vi "main.vi"() -> (5 "control":i32)   [LabVIEW 2014]
uses:
  <vilib>/Utility/miscctls.llb/LVPositionTypeDef.ctl
  Control 1.ctl
panel:
  out "Player2 energy":dbl
  out "Player1 skill":u8(slide) scale=0.0..100.0
  out "stop":bool
  out "Time(s)":dbl
  out "deliver2":T1
  out "deliver":T1
  out "player2":bool
  out "Position 2":T2
  out "control 2":i32
  out "test 2":i16
  out "player1":bool
  out "Position":T2
  out "test":i16
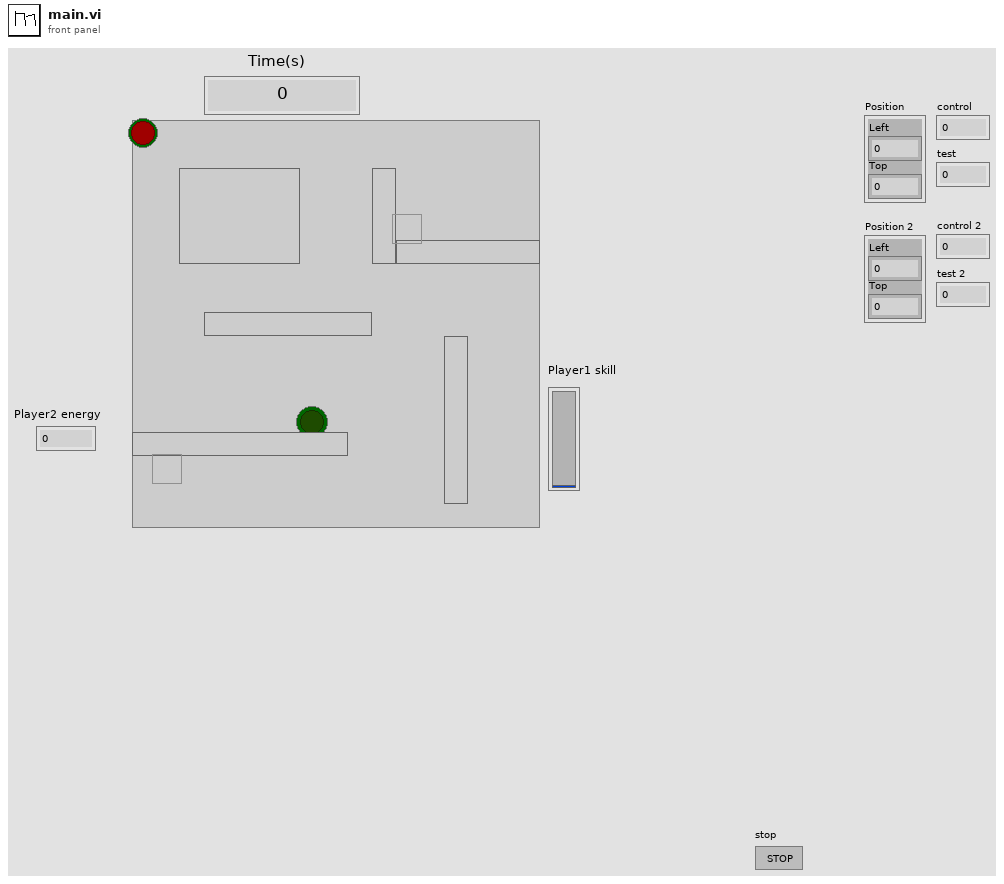
[diagram p1: front panel]
types:
  T1 = typedef "Control 1.ctl" = bool
  T2 = typedef "LVPositionTypeDef.ctl" = cluster{"Left":i32, "Top":i32}
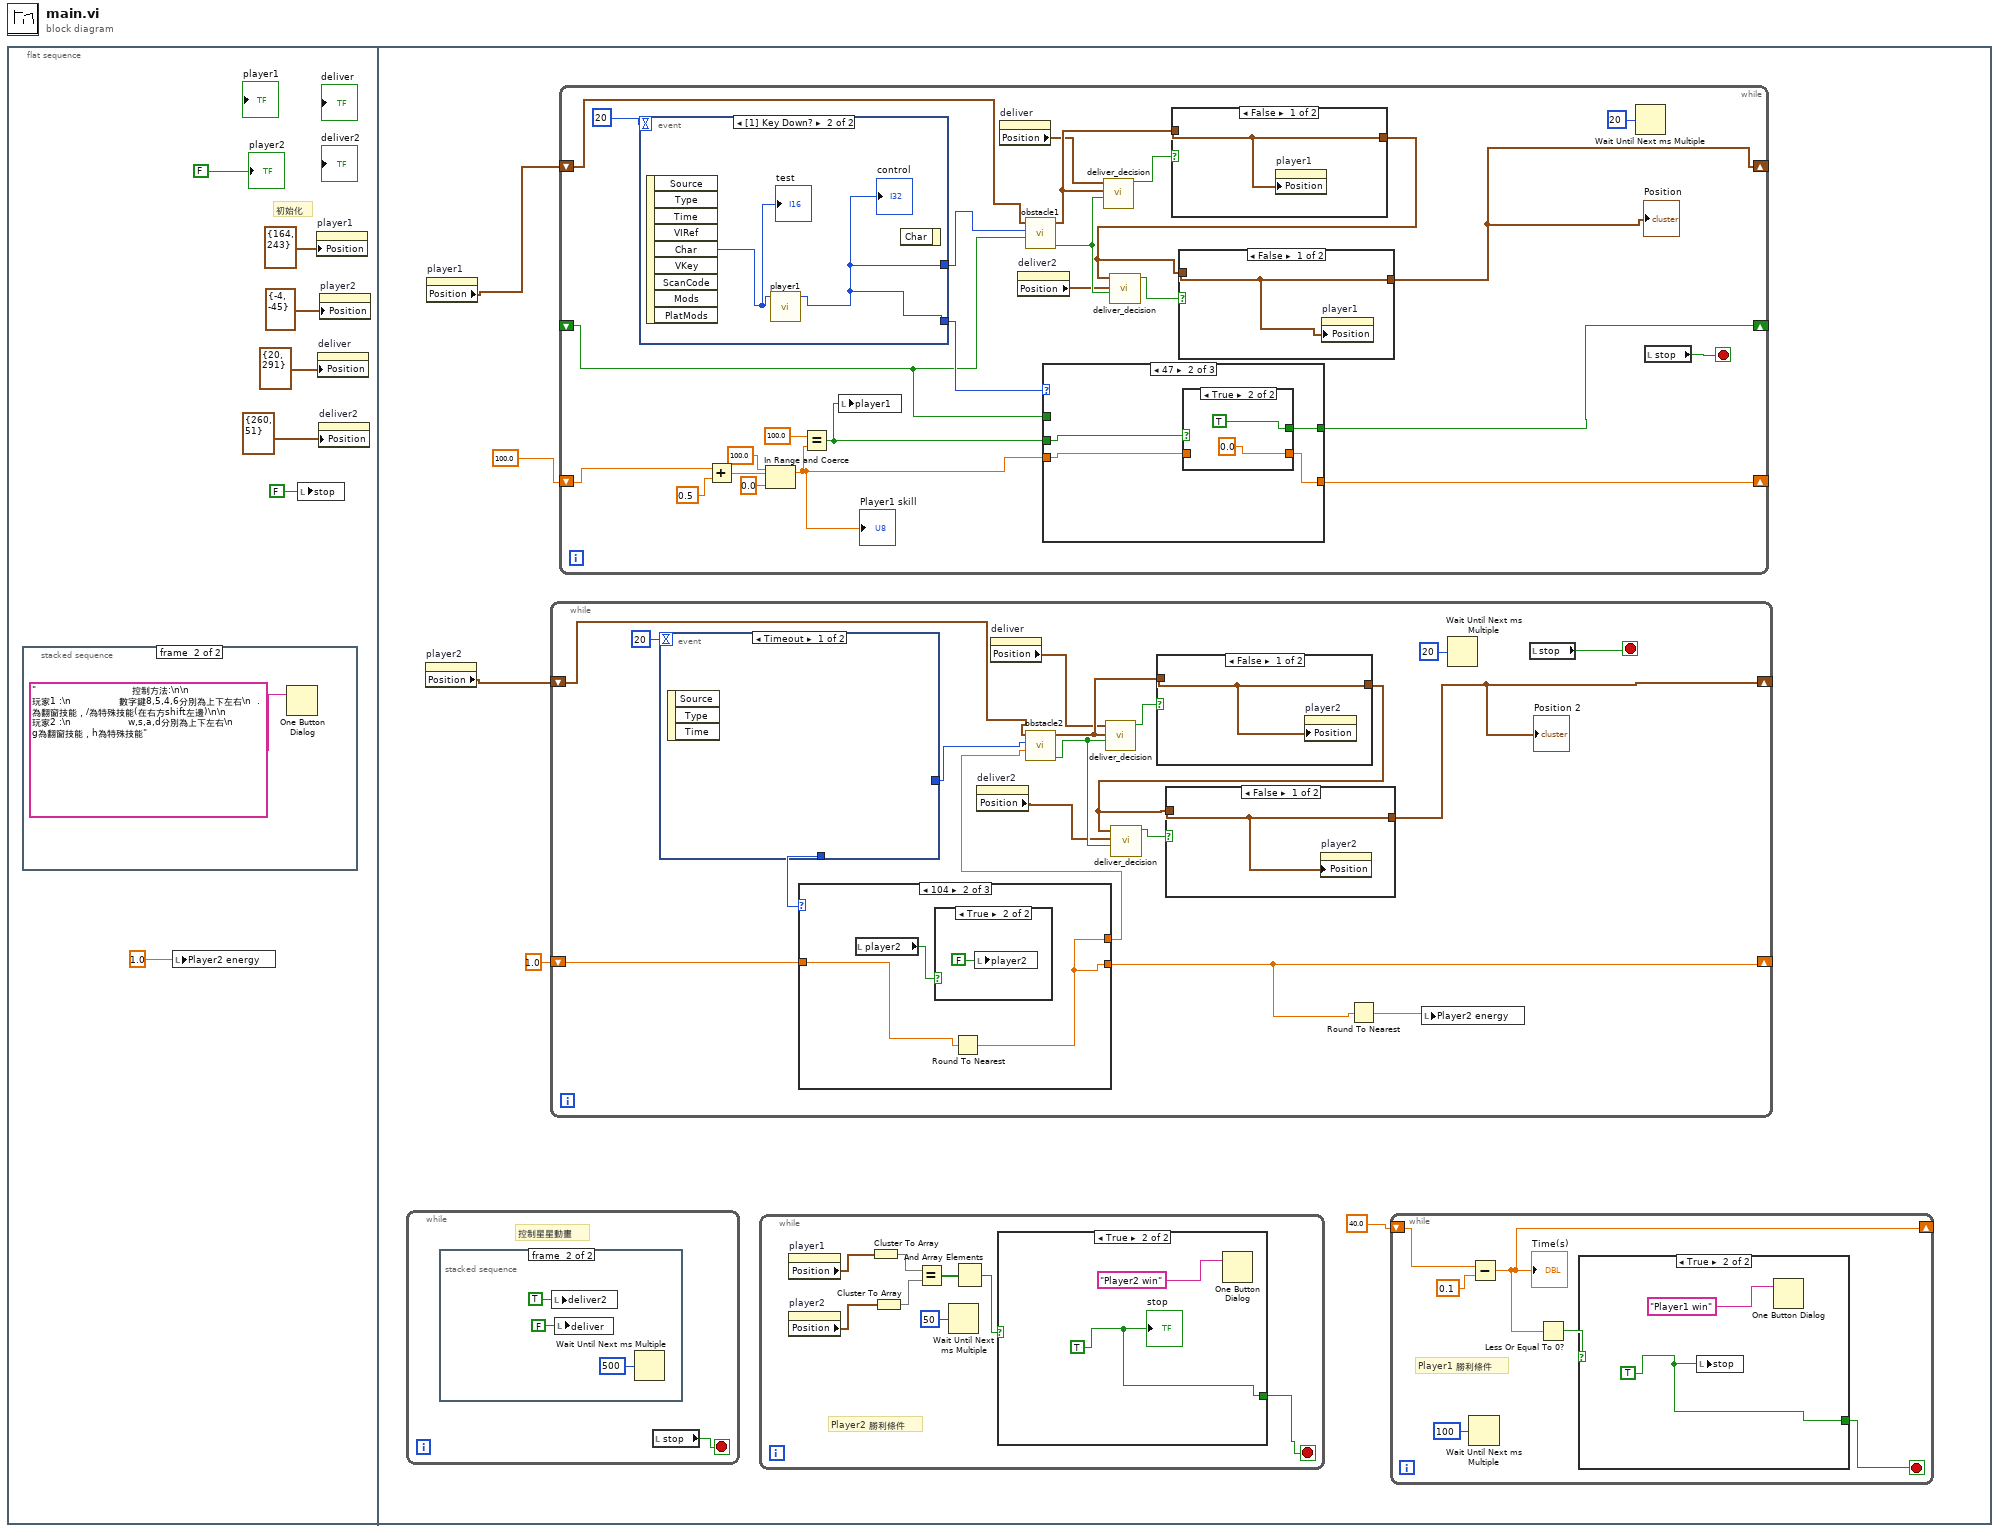
[diagram p0: block diagram]
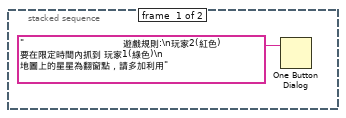
[diagram p2: hidden frame]
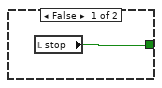
[diagram p3: hidden frame]
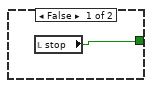
[diagram p4: hidden frame]
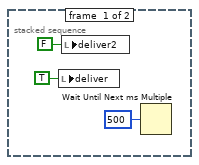
[diagram p5: hidden frame]
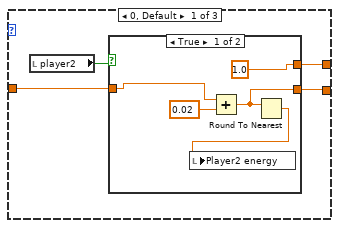
[diagram p6: hidden frame]
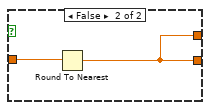
[diagram p7: hidden frame]
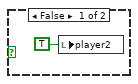
[diagram p8: hidden frame]
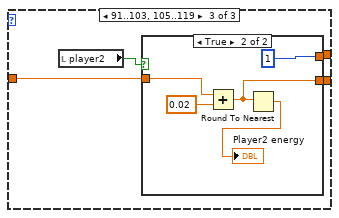
[diagram p9: hidden frame]
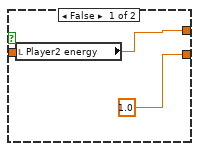
[diagram p10: hidden frame]
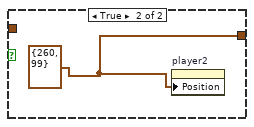
[diagram p11: hidden frame]
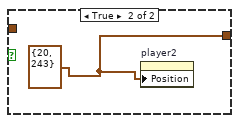
[diagram p12: hidden frame]
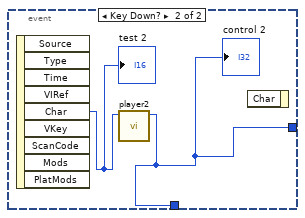
[diagram p13: hidden frame]
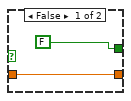
[diagram p15: hidden frame]
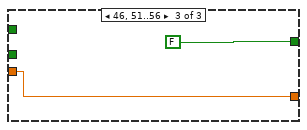
[diagram p16: hidden frame]
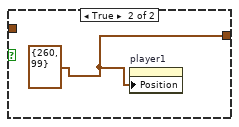
[diagram p17: hidden frame]
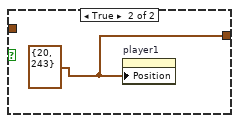
[diagram p18: hidden frame]
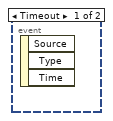
[diagram p19: hidden frame]
diagram:
  n1 = flat-sequence {
    frame #0 {
      # "初始化"
      n2 = stacked-sequence {
        frame #0 {
          n3 = One Button Dialog(message="                                 遊戲規則:\n玩家2(紅色) 要在限定時間內抓到 玩家1(綠色)\n       地圖上的星星為翻窗點，請多加利用") -> ()  [unwired: 1 in, 1 out]
        }
        frame #1 {
          n4 = One Button Dialog(message="                                控制方法:\n\n                                   玩家1 :\n                數字鍵8,5,4,6分別為上下左右\n  .為翻窗技能，/為特殊技能(在右方shift左邊)\n\n                                  玩家2 :\n                   w,s,a,d分別為上下左右\n               g為翻窗技能，h為特殊技能") -> ()  [unwired: 1 in, 1 out]
        }
      }
      n5 = local write "Player2 energy"(1.0 ("energy")) -> ()
      n6 = local write "stop"(FALSE ("stop 4")) -> ()
      n7 = property on="player1" class="Bool (strict)"("Position"=T2 {"Left"=164, "Top"=243}) -> ()  [unwired: 2 in, 2 out]
      n8 = property on="deliver" class="Bool (strict)"("Position"=T2 {"Left"=20, "Top"=291}) -> ()  [unwired: 2 in, 2 out]
      n9 = property on="deliver2" class="Bool (strict)"("Position"=T2 {"Left"=260, "Top"=51}) -> ()  [unwired: 2 in, 2 out]
      n10 = property on="player2" class="Bool (strict)"("Position"=T2 {"Left"=-4, "Top"=-45}) -> ()  [unwired: 2 in, 2 out]
      "player2" <- FALSE
    }
    frame #1 {
      n11 = while {
        stop <- w35 stop-if-true
        # "控制星星動畫"
        n12 = stacked-sequence {
          frame #0 {
            n13 = local write "deliver"(T1 TRUE ("deliver")) -> ()
            n14 = local write "deliver2"(T1 FALSE ("deliver2")) -> ()
            n15 = Wait Until Next ms Multiple(millisecond multiple=u32 500) -> ()  [unwired: 1 out]
          }
          frame #1 {
            n16 = local write "deliver2"(T1 TRUE ("deliver2")) -> ()
            n17 = local write "deliver"(T1 FALSE ("deliver")) -> ()
            n18 = Wait Until Next ms Multiple(millisecond multiple=u32 500) -> ()  [unwired: 1 out]
          }
        }
        n19 = local read "stop"() -> (w35:bool)
      }
      n20 = property on="player2" class="Bool (strict)"() -> ("Position"=w13:T2)  [unwired: 2 in, 2 out]
      n21 = property on="player1" class="Bool (strict)"() -> ("Position"=w14:T2)  [unwired: 2 in, 2 out]
      n22 = while {
        shift-right: [w51] -> _
        shift-left: w13 -> [w57]
        shift-right: [w43] -> _
        shift-left: 1.0 -> [w44]
        stop <- w48 stop-if-true
        n23 = event shown="[0] Timeout" {
          selector: _ -> [_ _]
          dyn-events: _ -> [_ _]
          timeout: 20 -> [_ _]
          tunnel: [_ w91] -> w58
          tunnel: [_ w91] -> w46
          event Timeout {
            n24 = event-data() -> ()  [unwired: 1 in, 3 out]
          }
          event Key Down? {
            n25 = event-data() -> ("Char"=w92:i16)  [unwired: 1 in, 8 out]
            "test 2" <- w92
            n26 = call "player2.vi"("Char"=w92) -> ("f"=w91:i32)  [unwired: 10 in]
            "control 2" <- w91
            n27 = event-data() -> ()  [unwired: 2 in, 1 out]
          }
        }
        n28 = case shown="104" w46 {
          tunnel: [w60 w71 w78] -> w45
          tunnel: [w62 w71 w77] -> w43
          tunnel: w44 -> [w63 w72 w76]
          frame 0, Default {
            n29 = local read "player2"() -> (w61:bool)
            n30 = case shown="True" w61 {
              tunnel: w63 -> [w67 w70]
              tunnel: [w64 w69] -> w62
              tunnel: [1.0 w69] -> w60
              frame True {
                n31 = Add(x=w67, y=0.02) -> (x+y=w64:dbl)
                n32 = Round To Nearest(number=w64) -> (nearest integer value=w65:dbl)
                n33 = local write "Player2 energy"(w65) -> ()
              }
              frame False {
                n34 = Round To Nearest(number=w70) -> (nearest integer value=w69:dbl)
              }
            }
          }
          frame 104 {
            n35 = local read "player2"() -> (w73:bool)
            n36 = case shown="True" w73 {
              frame False {
                n37 = local write "player2"(TRUE ("player2")) -> ()
              }
              frame True {
                n38 = local write "player2"(FALSE ("player2")) -> ()
              }
            }
            n39 = Round To Nearest(number=w72) -> (nearest integer value=w71:dbl)
          }
          frame 91..103, 105..119 {
            n40 = local read "player2"() -> (w79:bool)
            n41 = case shown="True" w79 {
              tunnel: [w81 1] -> w78
              tunnel: [1.0 w83] -> w77
              tunnel: w76 -> [_ w82]
              frame False {
                n42 = local read "Player2 energy"() -> (w81:dbl)
              }
              frame True {
                n43 = Add(x=w82, y=0.02) -> (x+y=w83:dbl)
                n44 = Round To Nearest(number=w83) -> (nearest integer value=→"Player2 energy":dbl)
              }
            }
          }
        }
        n45 = property on="deliver2" class="Bool (strict)"() -> ("Position"=w49:T2)  [unwired: 2 in, 2 out]
        n46 = property on="deliver" class="Bool (strict)"() -> ("Position"=w50:T2)  [unwired: 2 in, 2 out]
        n47 = call "obstacle2.vi"("Numeric"=w45, "f"=w58, "Position in"=w57) -> ("deliver"=w54:bool, "Position out"=w55:T2)  [unwired: 7 in]
        n48 = call "deliver_decision.vi"("deliver"=w54, "Position in"=w55, "Position"=w50) -> ("Boolean"=w56:bool)  [unwired: 8 in]
        n49 = case shown="False" w56 {
          tunnel: [w89 w90] -> w52
          tunnel: w55 -> [w89 _]
          frame False {
            n50 = property on="player2" class="Bool (strict)"("Position"=w89) -> ()  [unwired: 2 in, 2 out]
          }
          frame True {
            w90 = T2 {"Left"=20, "Top"=243} ("Position")
            n51 = property on="player2" class="Bool (strict)"("Position"=w90) -> ()  [unwired: 2 in, 2 out]
          }
        }
        n52 = call "deliver_decision.vi"("deliver"=w54, "Position in"=w49, "Position"=w52) -> ("Boolean"=w53:bool)  [unwired: 8 in]
        n53 = case shown="False" w53 {
          tunnel: [w87 w88] -> w51
          tunnel: w52 -> [w87 _]
          frame False {
            n54 = property on="player2" class="Bool (strict)"("Position"=w87) -> ()  [unwired: 2 in, 2 out]
          }
          frame True {
            w88 = T2 {"Left"=260, "Top"=99} ("Position")
            n55 = property on="player2" class="Bool (strict)"("Position"=w88) -> ()  [unwired: 2 in, 2 out]
          }
        }
        "Position 2" <- w51
        n56 = Round To Nearest(number=w43) -> (nearest integer value=w42:dbl)
        n57 = local write "Player2 energy"(w42) -> ()
        n58 = Wait Until Next ms Multiple(millisecond multiple=u32 20) -> ()  [unwired: 1 out]
        n59 = local read "stop"() -> (w48:bool)
      }
      n60 = while {
        shift-right: [w109] -> _
        shift-left: w14 -> [w116]
        shift-right: [w103] -> _
        shift-left: _ -> [w102]
        shift-right: [w101] -> _
        shift-left: 100.0 -> [w94]
        stop <- w106 stop-if-true
        n61 = event shown="[1] Key Down?" {
          selector: _ -> [_ _]
          dyn-events: _ -> [_ _]
          timeout: 20 -> [_ _]
          tunnel: [_ w134] -> w115
          tunnel: [_ w134] -> w104
          event Timeout {
            n62 = event-data() -> ()  [unwired: 1 in, 3 out]
          }
          event Key Down? {
            n63 = event-data() -> ("Char"=w135:i16)  [unwired: 1 in, 8 out]
            "test" <- w135
            n64 = call "player1.vi"("Char"=w135) -> ("f"=w134:i32)  [unwired: 10 in]
            "control" <- w134
            n65 = event-data() -> ()  [unwired: 2 in, 1 out]
          }
        }
        n66 = Add(x=w94, y=0.5) -> (x+y=w97:dbl)
        n67 = In Range and Coerce(upper limit=100.0, x=w97, lower limit=0.0) -> (coerced(x)=w95:dbl)  [unwired: 1 out]
        "Player1 skill" <- w95
        n68 = Equal?(x=100.0, y=w95) -> (x = y?=w93:bool)
        n69 = local write "player1"(w93) -> ()
        n70 = property on="deliver" class="Bool (strict)"() -> ("Position"=w108:T2)  [unwired: 2 in, 2 out]
        n71 = property on="deliver2" class="Bool (strict)"() -> ("Position"=w107:T2)  [unwired: 2 in, 2 out]
        n72 = call "obstacle1.vi"("Boolean"=w102, "f"=w115, "Position in"=w116) -> ("deliver"=w113:bool, "Position out"=w111:T2)  [unwired: 7 in]
        n73 = case shown="47" w104 {
          tunnel: [w118 w123 FALSE] -> w103
          tunnel: w102 -> [w118 _ _]
          tunnel: w95 -> [w119 w121 w128]
          tunnel: [w119 w122 w128] -> w101
          tunnel: w93 -> [_ w120 _]
          frame 0, Default {
          }
          frame 47 {
            n74 = case shown="True" w120 {
              tunnel: [FALSE TRUE] -> w123
              tunnel: w121 -> [w124 _]
              tunnel: [w124 0.0] -> w122
              frame False {
              }
              frame True {
              }
            }
          }
          frame 46, 51..56 {
          }
        }
        n75 = call "deliver_decision.vi"("deliver"=w113, "Position in"=w111, "Position"=w108) -> ("Boolean"=w114:bool)  [unwired: 8 in]
        n76 = case shown="False" w114 {
          tunnel: [w132 w133] -> w110
          tunnel: w111 -> [w132 _]
          frame False {
            n77 = property on="player1" class="Bool (strict)"("Position"=w132) -> ()  [unwired: 2 in, 2 out]
          }
          frame True {
            w133 = T2 {"Left"=20, "Top"=243} ("Position")
            n78 = property on="player1" class="Bool (strict)"("Position"=w133) -> ()  [unwired: 2 in, 2 out]
          }
        }
        n79 = call "deliver_decision.vi"("deliver"=w113, "Position in"=w107, "Position"=w110) -> ("Boolean"=w112:bool)  [unwired: 8 in]
        n80 = case shown="False" w112 {
          tunnel: [w130 w131] -> w109
          tunnel: w110 -> [w130 _]
          frame False {
            n81 = property on="player1" class="Bool (strict)"("Position"=w130) -> ()  [unwired: 2 in, 2 out]
          }
          frame True {
            w131 = T2 {"Left"=260, "Top"=99} ("Position")
            n82 = property on="player1" class="Bool (strict)"("Position"=w131) -> ()  [unwired: 2 in, 2 out]
          }
        }
        "Position" <- w109
        n83 = Wait Until Next ms Multiple(millisecond multiple=u32 20) -> ()  [unwired: 1 out]
        n84 = local read "stop"() -> (w106:bool)
      }
      n85 = while {
        stop <- w27 stop-if-true
        # "Player2 勝利條件"
        n86 = property on="player1" class="Bool (strict)"() -> ("Position"=w25:T2)  [unwired: 2 in, 2 out]
        n87 = property on="player2" class="Bool (strict)"() -> ("Position"=w24:T2)  [unwired: 2 in, 2 out]
        n88 = Cluster To Array(cluster=w25) -> (array=w31:i32[])
        n89 = Cluster To Array(cluster=w24) -> (array=w30:i32[])
        n90 = Equal?(x=w31, y=w30) -> (x = y?=w29:bool[])
        n91 = Wait Until Next ms Multiple(millisecond multiple=u32 50) -> ()  [unwired: 1 out]
        n92 = And Array Elements(Boolean array=w29) -> (logical AND=w28:bool)
        n93 = case shown="True" w28 {
          tunnel: [w32 w33] -> w27
          frame False {
            n94 = local read "stop"() -> (w32:bool)
          }
          frame True {
            w33 = TRUE
            n95 = One Button Dialog(message="Player2 win") -> ()  [unwired: 1 in, 1 out]
            "stop" <- w33
          }
        }
      }
      n96 = while {
        shift-right: [w16] -> _
        shift-left: 40.0 -> [w15]
        stop <- w17 stop-if-true
        # "Player1 勝利條件"
        n97 = Wait Until Next ms Multiple(millisecond multiple=u32 100) -> ()  [unwired: 1 out]
        n98 = Subtract(x=w15, y=0.1) -> (x-y=w16:dbl)
        "Time(s)" <- w16
        n99 = Less Or Equal To 0?(x=w16) -> (x <= 0?=w18:bool)
        n100 = case shown="True" w18 {
          tunnel: [w21 w22] -> w17
          frame False {
            n101 = local read "stop"() -> (w21:bool)
          }
          frame True {
            w22 = TRUE
            n102 = local write "stop"(w22) -> ()
            n103 = One Button Dialog(message="Player1 win") -> ()  [unwired: 1 in, 1 out]
          }
        }
      }
    }
  }
